vi "Get_Instrument_Instance.vi"(8 "error in (no error)":errorcluster, 10 "Factory_Data":variant) -> (0 "error out":errorcluster, 2 "Instruments":refnum<class "Abstract_Instrument.lvclass">[](array[class]))   [LabVIEW 2020, in "Abstract_Instrument.lvlib" / "Abstract_Instrument.lvclass"]
uses:
  Abstract_Instrument.lvclass
  Abstract_Instrument.lvclass/Abstract_Instrument.ctl
  <vilib>/MeasurementLink/MeasurementLink Session Management V1/Session Reservation/Session Reservation.lvclass/Session Reservation.ctl
  <vilib>/MeasurementLink/MeasurementLink Session Management V1/Session Reservation/Get Session Info - NSess .vi
  <vilib>/MeasurementLink/MeasurementLink Session Management V1/Session Reservation/Merge Invalid DVR Error.vi
  <vilib>/MeasurementLink/MeasurementLink Session Management V1/Session Reservation/Is DVR Valid.vi
  <vilib>/MeasurementLink/MeasurementLink Measurement Server/Helpers/Error Strings Global Internal.vi
  <vilib>/Utility/error.llb/Error Cluster From Error Code.vi
  <vilib>/MeasurementLink/MeasurementLink Session Management V1/Session Reservation/Session Reservation.lvclass
panel:
  in  "Abstract_Instrument in":refnum<class "Abstract_Instrument.lvclass">
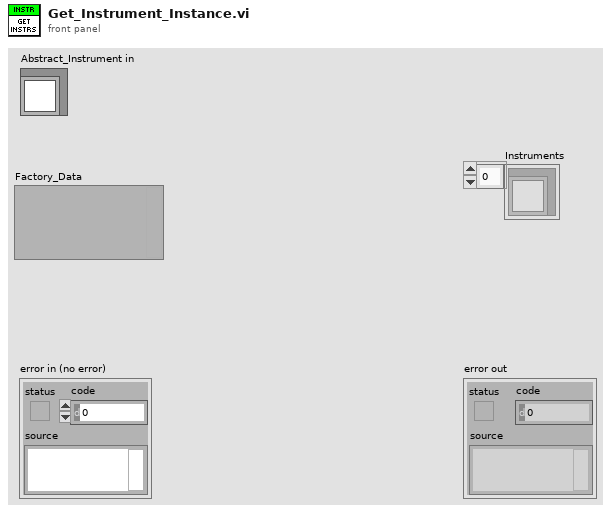
[diagram p1: front panel]
types:
  T1 = typedef "MeasurementLink Session Management Client.lvlib/ni_measurementlink_sessionmanagement_v1_SessionInformation.ctl" = cluster{"session":T2, "resource_name":string, "channel_list":string, "instrument_type_id":string, "session_exists":bool, "channel_mappings":T3[]}
  T2 = typedef "MeasurementLink Session Management Client.lvlib/nidevice_grpc_Session.ctl" = cluster{"name":string}
  T3 = typedef "MeasurementLink Session Management Client.lvlib/ni_measurementlink_sessionmanagement_v1_ChannelMapping.ctl" = cluster{"pin_or_relay_name":string, "site":i32, "channel":string, "multiplexer_resource_name":string, "multiplexer_route":string}
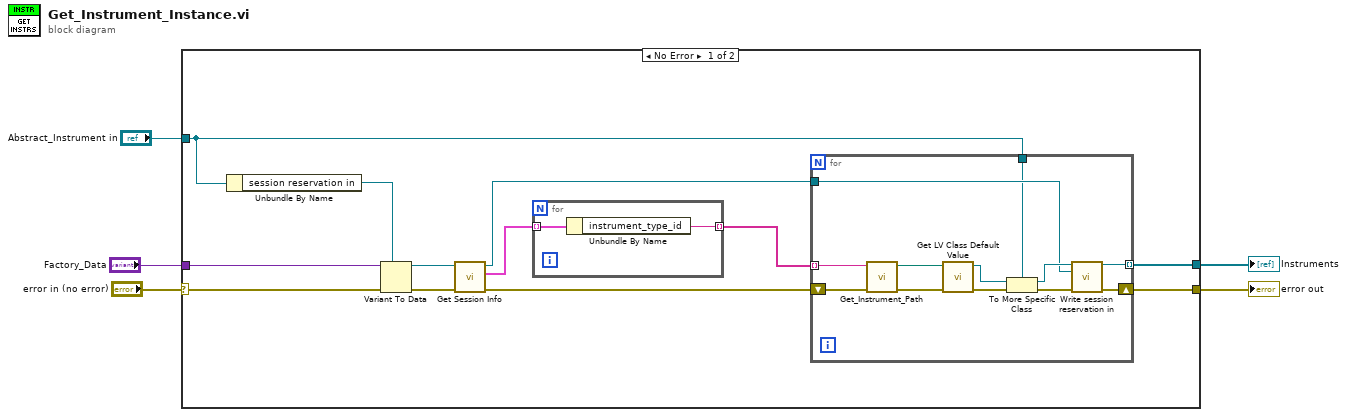
[diagram p0: block diagram]
diagram:
  n1 = case shown="No Error" "error in (no error)" {
    selector: "error in (no error)" -> [w16 w32]
    tunnel: [w12 w32] -> w4
    tunnel: "Abstract_Instrument in" -> [w8 _]
    tunnel: "Factory_Data" -> [w17 _]
    tunnel: [w9 _] -> w1
    frame No Error {
      n2 = Unbundle By Name(w8) -> ("session reservation in"=w7:refnum<class "Session Reservation.lvclass">)
      n3 = Variant To Data(error in=w16, type=w7, Variant=w17) -> (data=w14:refnum<class "Session Reservation.lvclass">, error out=w13:errorcluster)
      n4 = call-poly <vilib>:"Get Session Info.vi"("error in"=w13, "session reservation in"=w14) -> ("error out"=w11:errorcluster, "sessions info"=w15:T1[], "session reservation out"=w6:refnum<class "Session Reservation.lvclass">)  [unwired: 7 in]
      n5 = for {
        tunnel: [w31] -> w10 mode=indexing
        tunnel: w15 -> [w30] mode=indexing
        n6 = Unbundle By Name(w30) -> ("instrument_type_id"=w31:string)
      }
      n7 = for {
        shift-right: [w24] -> w12
        shift-left: w11 -> [w26]
        tunnel: w10 -> [w19] mode=indexing
        tunnel: [w22] -> w9 mode=indexing
        tunnel: w6 -> [w21]
        tunnel: w8 -> [w20]
        n8 = call "Get_Instrument_Path.vi"("error in (no error)"=w26, "instrument_type_id"=w19) -> ("error out"=w27:errorcluster, "InstrumentClassPath"=w18:path)  [unwired: 8 in]
        n9 = call <vilib>:"Get LV Class Default Value.vi"("error in (no error)"=w27, "class path"=w18) -> ("error out"=w29:errorcluster, "object"=w28:refnum<class>)  [unwired: 8 in]
        n10 = To More Specific Class(target class=w20, reference=w28, error in=w29) -> (specific class reference=w23:refnum<class "Abstract_Instrument.lvclass">, error out=w25:errorcluster)
        n11 = call-dynamic "Write session reservation in.vi"("AbstractDMM in"=w23, "MeasurementLink Session Management V1.lvlib:Session Reservation.lvclass"=w21, "error in (no error)"=w25) -> ("AbstractDMM out"=w22:refnum<class "Abstract_Instrument.lvclass">, "error out"=w24:errorcluster)  [unwired: 11 in]
      }
    }
    frame Error {
    }
  }
  "error out" <- w4
  "Instruments" <- w1
